vi "hardware_apply_settings.vi"(8 "error in (no error)":errorcluster, 11 "tt20 in":refnum<class "tt20.lvclass">) -> (0 "error out":errorcluster, 3 "tt20 out":refnum<class "tt20.lvclass">)   [LabVIEW 2015, in "tt20.lvclass"]
uses:
  tt20.lvclass
  detector/detector.lvclass
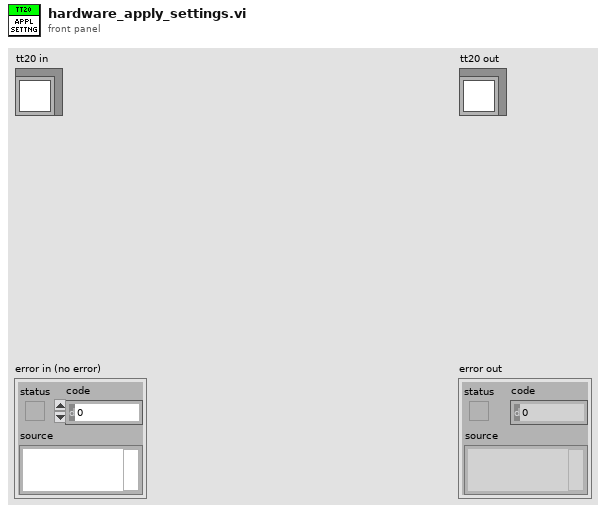
[diagram p1: front panel]
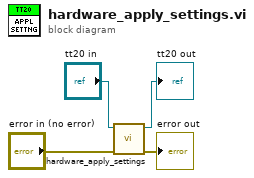
[diagram p0: block diagram]
diagram:
  n1 = call-parent "hardware_apply_settings.vi"("error in (no error)"="error in (no error)", "hardware in"="tt20 in") -> ("error out"=→"error out":errorcluster, "hardware out"=→"tt20 out":refnum<class "tt20.lvclass">)  [unwired: 8 in]
